vi "Get Logging Execution Time.vi"(8 "error in":errorcluster, 11 "timing ref":T1=18446744073709551615 format="%.0x") -> (0 "error out":errorcluster, 2 "logging execution time ref":T1 format="%.0x", 3 "timing ref out":T1 format="%.0x")   [LabVIEW 2024, in "AIM ARINC 429 Scripting.lvlib"]
doc: "Returns true if logging is enabled."
uses:
  AIM ARINC 429 Scripting.lvlib
  <vilib>/NI VeriStand/Custom Device API/Custom Device Item Ref.ctl
  Constants.vi
  <vilib>/NI VeriStand/Custom Device Tools/Custom Device Utility Library/NI VeriStand - Search for Item by Name.vi
  <vilib>/NI VeriStand/Custom Device Tools/Custom Device Utility Library/Custom Device Utility Library.lvlib
  <vilib>/NI VeriStand/Custom Device API/Custom Device API.lvlib
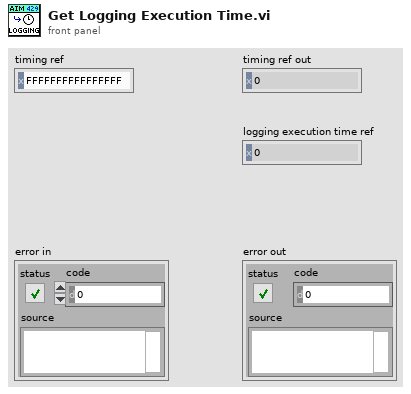
[diagram p1: front panel]
types:
  T1 = typedef "Custom Device API.lvlib/Custom Device Item Ref.ctl" = u64
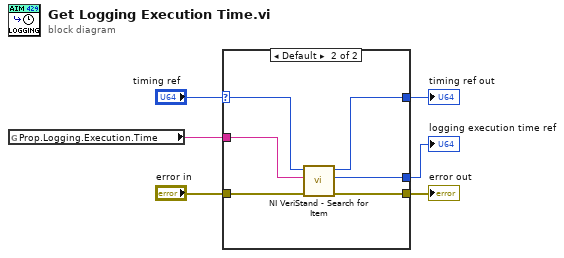
[diagram p0: block diagram]
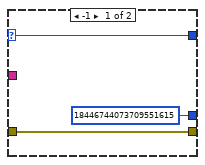
[diagram p2: hidden frame]
diagram:
  n1 = global read "Constants.vi" "Prop.Logging.Execution.Time"() -> (w6:string)
  n2 = case shown="Default" "timing ref" {
    selector: "timing ref" -> [w7 w11]
    tunnel: w6 -> [_ w15]
    tunnel: "error in" -> [w9 w14]
    tunnel: [w7 w13] -> w4
    tunnel: [w9 w12] -> w3
    tunnel: [T1 18446744073709551615 ("Item Ref") w10] -> w1
    frame -1 {
    }
    frame Default {
      n3 = call-poly <vilib>:"NI VeriStand - Search for Item.vi"("error in"=w14, "Item Name"=w15, "Section Ref in"=w11) -> ("error out"=w12:errorcluster, "Item Ref"=w10:T1, "Section Ref out"=w13:T1)  [unwired: 5 in, 1 out]
    }
  }
  "error out" <- w3
  "timing ref out" <- w4
  "logging execution time ref" <- w1
